vi "Drop Message.vi"(11 "Message in":refnum<class "Message.lvclass">) -> ()   [LabVIEW 2013, in "Actor Framework.lvlib" / "Message.lvclass"]
doc: "(<B>Filename</B>: Actor Framework.lvlib:Message.lvclass:Drop Message.vi)\n\nWrapper for Drop Message Core.vi"
uses:
  <vilib>/ActorFramework/Message/Message.lvclass
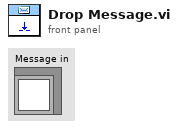
[diagram p1: front panel]
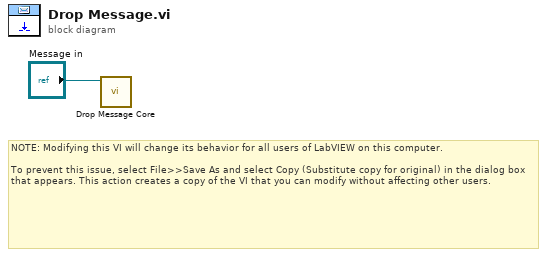
[diagram p0: block diagram]
diagram:
  # "NOTE: Modifying this VI will change its behavior for all users of LabVIEW on this computer.\n\nTo prevent this issue, select File>>Save As and select Copy (Substitute copy for original) in the dialog box that appears. This action creates a copy of the VI that you can modify without affecting other users."
  n1 = call-dynamic "Drop Message Core.vi"("Message in"="Message in") -> ()  [unwired: 11 in]
